vi "Diff_Drive_System_Set_AutoTuneCO_Offset.vi"(9 "Right CO Offset":dbl, 11 "Left CO Offset":dbl) -> ()   [LabVIEW 2019]
uses:
  Diff_Drive_System_Globals.vi
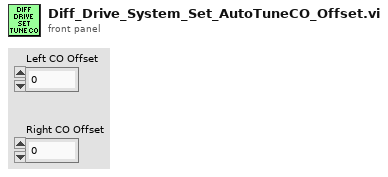
[diagram p1: front panel]
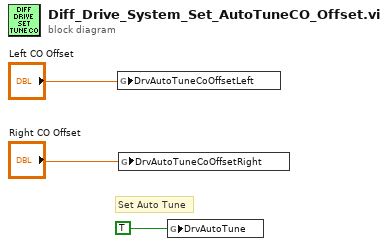
[diagram p0: block diagram]
diagram:
  # "Set Auto Tune"
  n1 = global write "Diff_Drive_System_Globals.vi" "DrvAutoTuneCoOffsetLeft"("Left CO Offset") -> ()
  n2 = global write "Diff_Drive_System_Globals.vi" "DrvAutoTuneCoOffsetRight"("Right CO Offset") -> ()
  n3 = global write "Diff_Drive_System_Globals.vi" "DrvAutoTune"(TRUE ("AutoTune")) -> ()
